vi "Parse.vi"(8 "error in (no error)":errorcluster, 11 "PathCommands.LineTo in":refnum<class "PathCommands.LineTo.lvclass">) -> (0 "error out":errorcluster, 3 "PathCommands.LineTo out":refnum<class "PathCommands.LineTo.lvclass">)   [LabVIEW 2019, in "PathCommands.LineTo.lvclass"]
uses:
  PathCommands.LineTo.lvclass
  <vilib>/Utility/error.llb/whitespace.ctl
  PathCommands/Point.ctl
  PathCommands/PathCommands.lvclass
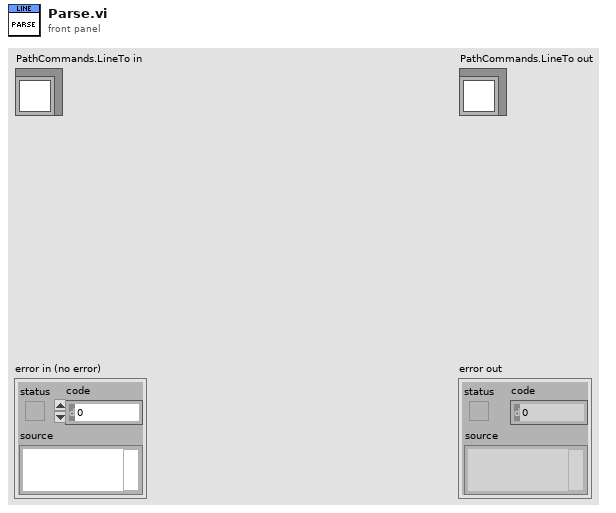
[diagram p1: front panel]
types:
  T1 = typedef "whitespace.ctl" = u16
  T2 = typedef "PathCommands.lvclass/Point.ctl" = cluster{"X":dbl, "Y":dbl}
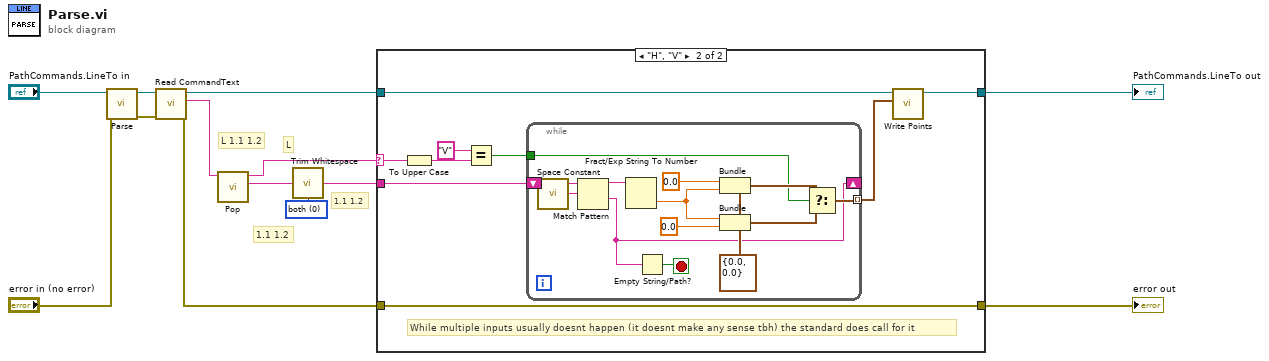
[diagram p0: block diagram]
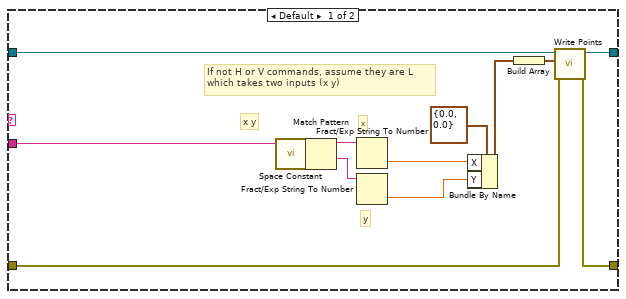
[diagram p2: hidden frame]
diagram:
  w1 = T1 0 items=["both", "start of string", "end of string"] ("location (both)")
  # "1.1 1.2"
  # "1.1 1.2"
  # "L"
  # "L 1.1 1.2"
  n1 = call-parent "Parse.vi"("error in (no error)"="error in (no error)", "PathCommands in"="PathCommands.LineTo in") -> ("error out"=w10:errorcluster, "PathCommands out"=w11:refnum<class "PathCommands.LineTo.lvclass">)  [unwired: 8 in]
  n2 = call-dynamic "Read CommandText.vi"("error in (no error)"=w10, "PathCommands in"=w11) -> ("error out"=w4:errorcluster, "CommandText"=w9:string, "PathCommands out"=w5:refnum<class "PathCommands.LineTo.lvclass">)  [unwired: 7 in]
  n3 = call "Pop.vi"("Command Text"=w9) -> ("Command Info"=w7:string, "Command Type"=w8:string)  [unwired: 9 in]
  n4 = call <vilib>:"Trim Whitespace.vi"("string"=w7, "location (both)"=w1) -> ("trimmed string"=w2:string)
  n5 = case shown="\"H\", \"V\"" w8 {
    selector: w8 -> [_ w34]
    tunnel: w2 -> [w26 w31]
    tunnel: [w22 w30] -> w6
    tunnel: w5 -> [w21 w29]
    tunnel: w4 -> [w15 w35]
    tunnel: [w16 w35] -> w3
    frame Default {
      # "y"
      # "x"
      # "x y"
      # "If not H or V commands, assume they are L\nwhich takes two inputs (x y)"
      n6 = call <vilib>:"Space Constant.vi"() -> ("String"=w25:string)
      n7 = Match Pattern(string=w26, regular expression=w25) -> (before substring=w23:string, after substring=w24:string)  [unwired: 1 in, 2 out]
      n8 = Fract/Exp String To Number(string=w23) -> (number=w20:dbl)  [unwired: 3 in, 1 out]
      n9 = Fract/Exp String To Number(string=w24) -> (number=w19:dbl)  [unwired: 3 in, 1 out]
      n10 = Bundle By Name(cluster=T2 {"X"=0.0, "Y"=0.0} ("Point"), "X"=w20, "Y"=w19) -> (w17:T2)
      n11 = Build Array(w17) -> (w18:T2[])
      n12 = call-dynamic "Write Points.vi"("error in (no error)"=w15, "Points"=w18, "PathCommands in"=w21) -> ("error out"=w16:errorcluster, "PathCommands out"=w22:refnum<class "PathCommands.LineTo.lvclass">)  [unwired: 7 in]
    }
    frame "H", "V" {
      # "While multiple inputs usually doesnt happen (it doesnt make any sense tbh) the standard does call for it"
      n13 = To Upper Case(1:w34) -> (0:w33:string)
      n14 = Equal?(x="V", y=w33) -> (x = y?=w28:bool)
      n15 = while {
        tunnel: w28 -> [w42]
        tunnel: [w41] -> w27 mode=indexing
        shift-right: [w36] -> _
        shift-left: w31 -> [w39]
        stop <- w37 stop-if-true
        w48 = T2 {"X"=0.0, "Y"=0.0} ("Point")
        n16 = call <vilib>:"Space Constant.vi"() -> ("String"=w38:string)
        n17 = Match Pattern(string=w39, regular expression=w38) -> (before substring=w40:string, after substring=w36:string)  [unwired: 1 in, 2 out]
        n18 = Fract/Exp String To Number(string=w40) -> (number=w47:dbl)  [unwired: 3 in, 1 out]
        n19 = Empty String/Path?(string/path=w36) -> (empty?=w37:bool)
        n20 = Bundle(cluster=w48, "X"=0.0, "Y"=w47) -> (w44:T2)
        n21 = Bundle(cluster=w48, "X"=w47, "Y"=0.0) -> (w43:T2)
        n22 = Select(t=w44, s=w42, f=w43) -> (s? t:f=w41:T2)
      }
      n23 = call-dynamic "Write Points.vi"("Points"=w27, "PathCommands in"=w29) -> ("PathCommands out"=w30:refnum<class "PathCommands.LineTo.lvclass">)  [unwired: 8 in, 1 out]
    }
  }
  "error out" <- w3
  "PathCommands.LineTo out" <- w6
